vi "Turret.vi"() -> ()   [LabVIEW 2019]
uses:
  refnums.vi
  TAI_Servo.vi
  658ec7b6-7da6-42d7-bb00-7c97577ff0d5.vi
  sensors.vi
panel:
  in  "Servo_Commanded_Angle":dbl
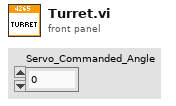
[diagram p1: front panel]
types:
  T1 = typedef "WPI_ServoDeviceRef.ctl" = cluster{"DeviceStatus":errorcluster, "PWM Channel":T2, "DeadBand":T3}
  T2 = typedef "FPGA_DIOPWMChannel.ctl" = enum8{"PWM 0", "PWM 1", "PWM 2", "PWM 3", "PWM 4", "PWM 5", "PWM 6", "PWM 7", "PWM 8", "PWM 9", "PWM MXP 0", "PWM MXP 1", "PWM MXP 2", "PWM MXP 3", "PWM MXP 4", "PWM MXP 5", "PWM MXP 6", "PWM MXP 7", "PWM MXP 8", "PWM MXP 9", "Invalid"}
  T3 = typedef "WPI_PWMDeadband.ctl" = cluster{"Name":string, "maxPositivePwm":i32, "minPositivePwm":i32, "centerPwm":i32, "maxNegativePwm":i32, "minNegativePwm":i32, "angularRange":u16}
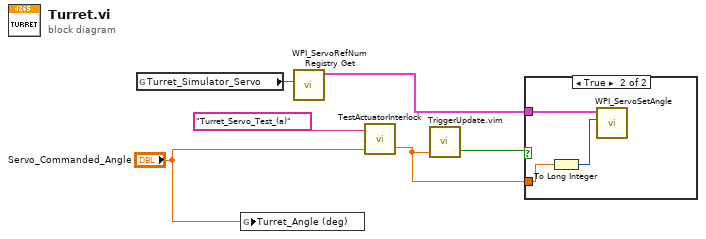
[diagram p0: block diagram]
diagram:
  n1 = global read "refnums.vi" "Turret_Simulator_Servo"() -> (w5:string)
  n2 = global write "sensors.vi" "Turret_Angle (deg)"("Servo_Commanded_Angle") -> ()
  n3 = call <vilib>:"WPI_ServoRefNum Registry Get.vi"("refnum name"=w5) -> ("ServoDeviceRef"=w4:T1)  [unwired: 9 in, 1 out]
  n4 = call-poly "TestActuatorInterlock.vi"("Normal Output"="Servo_Commanded_Angle", "Actuator Name"="Turret_Servo_Test_(a)") -> ("Interlock Output"=w3:dbl)  [unwired: 1 in, 1 out]
  n5 = call "TriggerUpdate.vim"("Trigger"=w3) -> ("Update"=w6:bool)  [unwired: 2 in]
  n6 = case shown="True" w6 {
    tunnel: w3 -> [_ w7]
    tunnel: w4 -> [_ w9]
    frame False {
    }
    frame True {
      n7 = To Long Integer(number=w7) -> (32bit integer=w8:i32)
      n8 = call <vilib>:"WPI_ServoSetAngle.vi"("Angle"=w8, "ServoDeviceRef"=w9) -> ()  [unwired: 8 in, 2 out]
    }
  }
